vi "LJU3_meas_v.vi"(5 "channel_list":i32[](array[numeric]), 6 "n_avg":i32=1000, 7 "IOTypes":string[](array[string]), 8 "error in":errorcluster, 11 "handle in":i32) -> (0 "error out":errorcluster, 1 "array_voltage":dbl[](array[numeric]), 3 "handle out":i32, 4 "status":bool=TRUE)   [LabVIEW 2019]
uses:
  <vilib>/Analysis/baseanly.llb/Mean (DBL).vi
  <vilib>/Analysis/NI_AALBase.lvlib
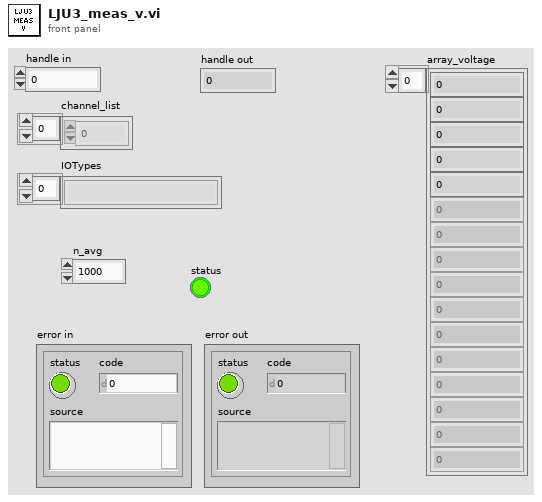
[diagram p1: front panel]
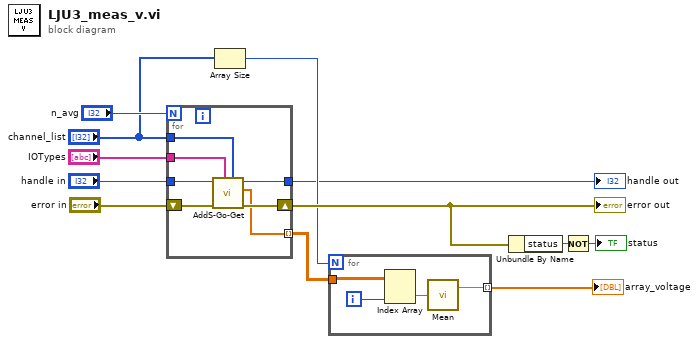
[diagram p0: block diagram]
diagram:
  n1 = for {
    N: "n_avg" -> [_]
    tunnel: [w13] -> w7 mode=indexing
    shift-right: [w18] -> w11
    shift-left: "error in" -> [w19]
    tunnel: "handle in" -> [w17]
    tunnel: [w16] -> w3
    tunnel: "IOTypes" -> [w15]
    tunnel: "channel_list" -> [w14]
    n2 = call "AddS-Go-Get.vi"("Channels"=w14, "IOTypes"=w15, "error in"=w19, "Handle In"=w17) -> ("error out"=w18:errorcluster, "Values Read"=w13:dbl[], "Handle Out"=w16:i32)  [unwired: 5 in]
  }
  "error out" <- w11
  "handle out" <- w3
  n3 = Array Size(array="channel_list") -> (size(s)=w6:i32)
  n4 = for {
    N: w6 -> [_]
    tunnel: w7 -> [w23]
    tunnel: [w20] -> w5 mode=indexing
    i -> [w22]
    n5 = Index Array(array=w23, index (col)=w22) -> (element=w21:dbl[])  [unwired: 1 in]
    n6 = call-poly <vilib>:"Mean.vi"("X"=w21) -> ("mean"=w20:dbl)  [unwired: 1 out]
  }
  "array_voltage" <- w5
  n7 = Unbundle By Name(w11) -> ("status"=w10:bool)
  n8 = Not(x=w10) -> (.not. x?=→"status":bool)
